vi "Initialize Buffer Data.vi"(8 "error in (no error)":errorcluster, 9 "Max Buffer Size [bytes] (20M)":i64=20000000, 10 "Buffer Size":i64, 11 "Channel Count":i32) -> (0 "error out":errorcluster, 3 "Buffer Data":T1)   [LabVIEW 2012, in "Triggered Log.lvclass"]
doc: "Initialize the log data buffer according to the specified buffer size (depth) and number of channels. Each channel's data is represented as a row in the buffer, where each column is a data point for that channel."
uses:
  Triggered Log.lvclass
  Buffer Data.ctl
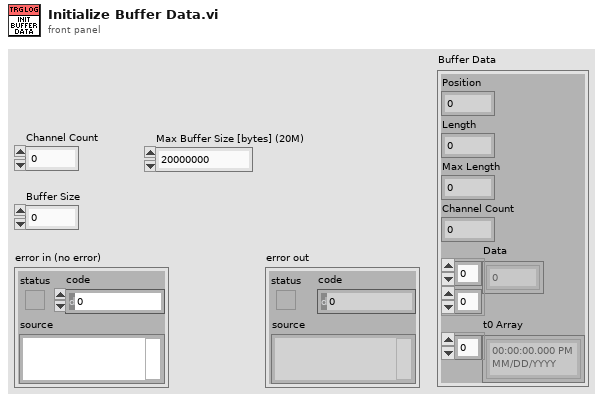
[diagram p1: front panel]
types:
  T1 = typedef "Triggered Log.lvclass/Buffer Data.ctl" = cluster{"Position":i32, "Length":i32, "Max Length":i32, "Channel Count":i32, "Data":dbl[][], "t0 Array":timestamp[]}
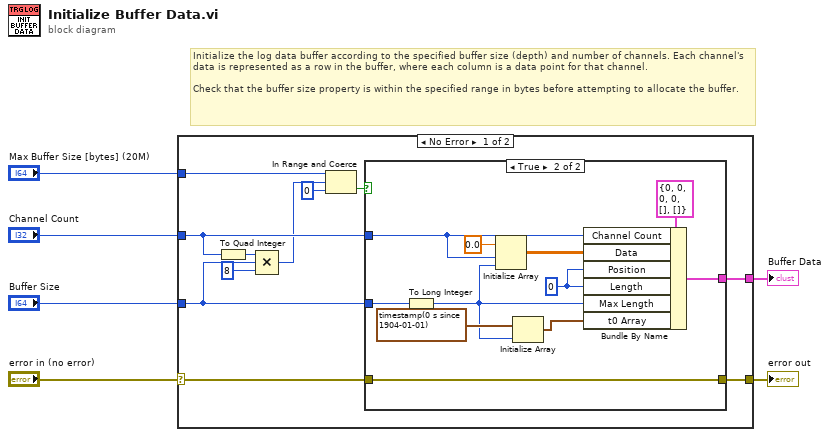
[diagram p0: block diagram]
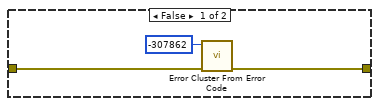
[diagram p2: hidden frame]
diagram:
  # "Initialize the log data buffer according to the specified buffer size (depth) and number of channels. Each channel's data is represented as a row in the buffer, where each column is a data point for that channel.\n\nCheck that the buffer size property is within the specified range in bytes before attempting to allocate the buffer."
  n1 = case shown="No Error" "error in (no error)" {
    selector: "error in (no error)" -> [w13 w32]
    tunnel: [w14 w32] -> w2
    tunnel: [w17 _] -> w3
    tunnel: "Channel Count" -> [w12 _]
    tunnel: "Buffer Size" -> [w10 _]
    tunnel: "Max Buffer Size [bytes] (20M)" -> [w8 _]
    frame No Error {
      n2 = To Quad Integer(1:w12) -> (0:w9:i64)
      n3 = Compound Arithmetic op=MULTIPLY(w9, w10, i64 8 ("value")) -> (w11:i64)
      n4 = In Range and Coerce(upper limit=w8, x=w11, lower limit=i64 0) -> (In Range?=w15:bool)  [unwired: 1 out]
      n5 = case shown="True" w15 {
        tunnel: [_ w28] -> w17
        tunnel: w12 -> [_ w26]
        tunnel: [w18 w25] -> w14
        tunnel: w13 -> [w19 w25]
        tunnel: w10 -> [_ w24]
        frame False {
          n6 = call <vilib>:"Error Cluster From Error Code.vi"("error in (no error)"=w19, "error code (0)"=-307862) -> ("error out"=w18:errorcluster)  [unwired: 7 in]
        }
        frame True {
          w29 = 0 ("Last")
          n7 = To Long Integer(number=w24) -> (32bit integer=w22:i32)
          n8 = Initialize Array(0.0 ("element"), w26, w22) -> (w30:dbl[][])
          n9 = Initialize Array(timestamp(0 s since 1904-01-01), w22) -> (w21:timestamp[])
          n10 = Bundle By Name(cluster=T1 {"Position"=0, "Length"=0, "Max Length"=0, "Channel Count"=0, "Data"=[], "t0 Array"=[]} ("Buffer Data"), "Channel Count"=w26, "Data"=w30, "Position"=w29, "Length"=w29, "Max Length"=w22, "t0 Array"=w21) -> (w28:T1)
        }
      }
    }
    frame Error {
    }
  }
  "Buffer Data" <- w3
  "error out" <- w2
